vi "Destroy Front Panel Events.vi"(8 "error in (no error)":errorcluster, 11 "Viewer in":refnum<class "Viewer.lvclass">) -> (0 "error out":errorcluster, 3 "Viewer out":refnum<class "Viewer.lvclass">)   [LabVIEW 2015, in "Viewer.lvlib" / "Viewer.lvclass"]
uses:
  Viewer.lvclass
  UI Window/UI Window.lvclass
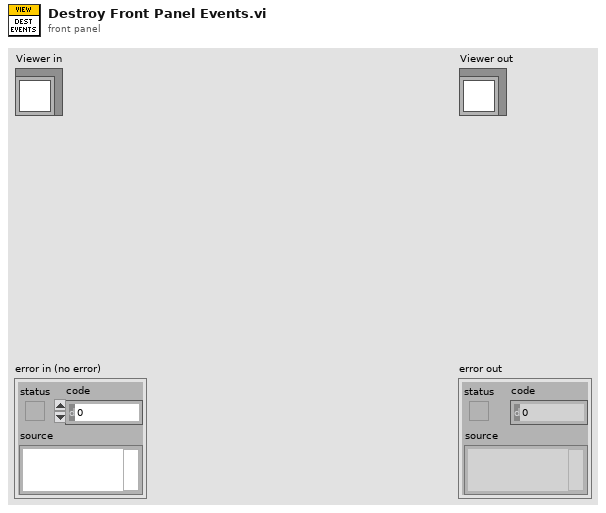
[diagram p1: front panel]
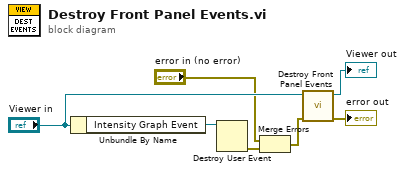
[diagram p0: block diagram]
diagram:
  n1 = Unbundle By Name("Viewer in") -> ("Intensity Graph Event"=w4:refnum<user-event>)
  n2 = Destroy User Event(user event=w4) -> (error out=w3:errorcluster)  [unwired: 1 in]
  n3 = Merge Errors("error in (no error)", w3) -> (w1:errorcluster)
  n4 = call-parent "Destroy Front Panel Events.vi"("error in (no error)"=w1, "UI Window in"="Viewer in") -> ("error out"=→"error out":errorcluster, "UI Window out"=→"Viewer out":refnum<class "Viewer.lvclass">)  [unwired: 8 in]
